vi "Driver Scaling.vi"(1 "Scaling Type":T1=enum."RSVP5", 2 "x":dbl) -> (0 "y":dbl)   [LabVIEW 2020]
uses:
  Types/Scaling Types.ctl
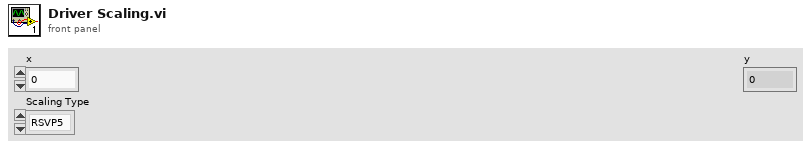
[diagram p1: front panel]
types:
  T1 = typedef "Scaling Types.ctl" = enum16{"Linear", "Square", "Cube", "RSVP5"}
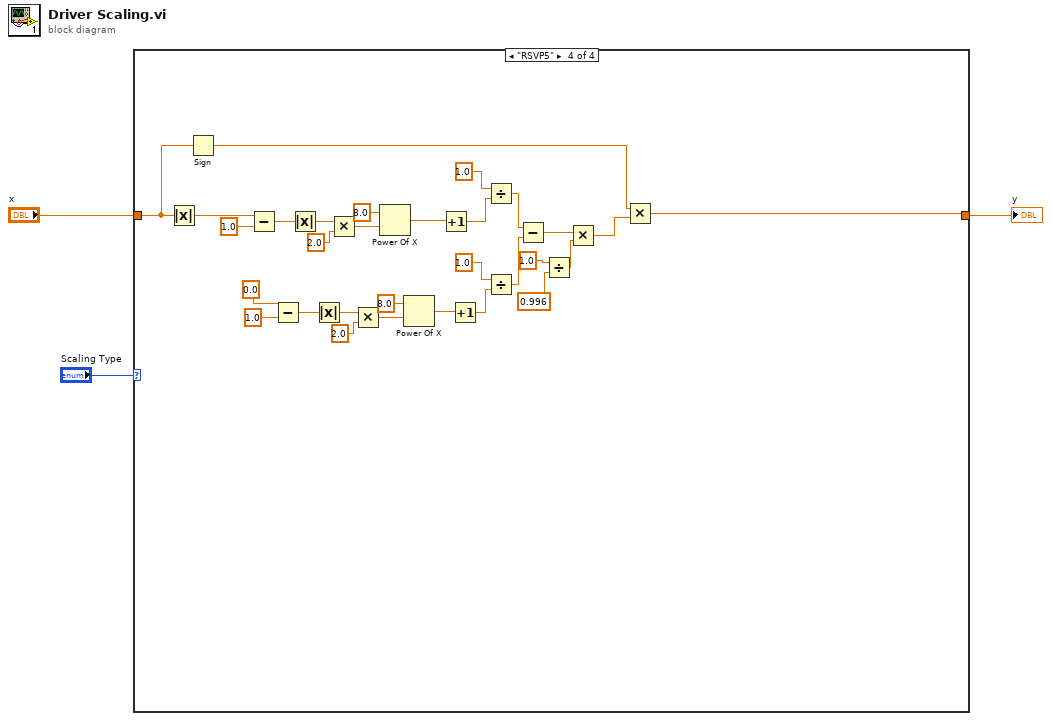
[diagram p0: block diagram]
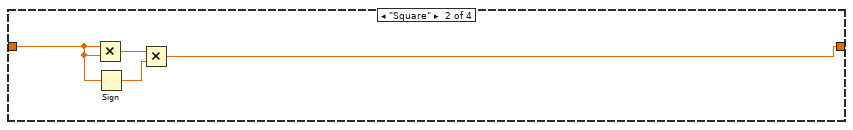
[diagram p3: hidden frame]
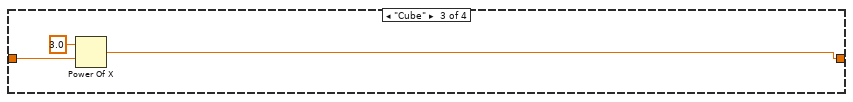
[diagram p4: hidden frame]
diagram:
  n1 = case shown="\"RSVP5\"" "Scaling Type" {
    tunnel: "x" -> [w4 w7 w11 w18]
    tunnel: [w4 w5 w9 w16] -> w2
    frame "Linear", Default {
    }
    frame "Square" {
      n2 = Multiply(x=w7, y=w7) -> (x*y=w8:dbl)
      n3 = Sign(1:w7) -> (0:w6:dbl)
      n4 = Multiply(x=w8, y=w6) -> (x*y=w5:dbl)
    }
    frame "Cube" {
      n5 = Power Of X(1:w11, 2:3.0 ("y")) -> (0:w9:dbl)
    }
    frame "RSVP5" {
      n6 = Absolute Value(x=w18) -> (abs(x)=w20:dbl)
      n7 = Sign(1:w18) -> (0:w17:dbl)
      n8 = Subtract(x=w20, y=1.0) -> (x-y=w39:dbl)
      n9 = Subtract(x=0.0 ("y"), y=1.0) -> (x-y=w32:dbl)
      n10 = Absolute Value(x=w39) -> (abs(x)=w38:dbl)
      n11 = Absolute Value(x=w32) -> (abs(x)=w31:dbl)
      n12 = Multiply(x=w38, y=2.0 ("x")) -> (x*y=w36:dbl)
      n13 = Multiply(x=w31, y=2.0 ("x")) -> (x*y=w29:dbl)
      n14 = Power Of X(1:w36, 2:8.0 ("y")) -> (0:w15:dbl)
      n15 = Power Of X(1:w29, 2:8.0 ("y")) -> (0:w13:dbl)
      n16 = Increment(x=w15) -> (x+1=w14:dbl)
      n17 = Increment(x=w13) -> (x+1=w12:dbl)
      n18 = Divide(x=1.0, y=w14) -> (x/y=w26:dbl)
      n19 = Divide(x=1.0, y=w12) -> (x/y=w25:dbl)
      n20 = Subtract(x=w26, y=w25) -> (x-y=w24:dbl)
      n21 = Divide(x=1.0, y=0.996) -> (x/y=w21:dbl)
      n22 = Multiply(x=w24, y=w21) -> (x*y=w19:dbl)
      n23 = Multiply(x=w17, y=w19) -> (x*y=w16:dbl)
    }
  }
  "y" <- w2
